vi "ex_2_test.vi"() -> ()   [LabVIEW 2020]
panel:
  out "Counter":i32
  in  "stop":bool
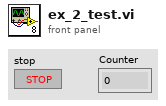
[diagram p1: front panel]
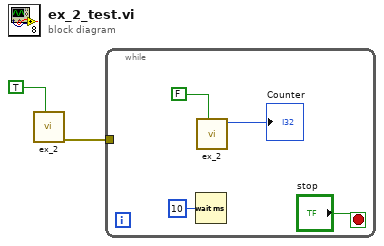
[diagram p0: block diagram]
diagram:
  n1 = call "ex_2.vi"("Reset (T)/Count (F)"=TRUE) -> ("error out"=w1:errorcluster)  [unwired: 9 in, 1 out]
  n2 = while {
    tunnel: w1 -> [_]
    stop <- "stop" stop-if-true
    n3 = Wait (ms)(milliseconds to wait=u32 10) -> ()  [unwired: 1 out]
    n4 = call "ex_2.vi"("Reset (T)/Count (F)"=FALSE) -> ("Counter"=→"Counter":i32)  [unwired: 9 in, 1 out]
  }
